vi "ULSIFD.vi"(0 "IFD in":refnum<class "IFD.lvclass">, 1 "ROI":cluster{"X1":sgl, "X2":sgl, "Y1":sgl, "Y2":sgl}={"X1"=0.0, "X2"=1.0, "Y1"=0.0, "Y2"=1.0}, 2 "General Info":T6={"CCD Model Num"="V10E", "Exposure time(ms)"=10.0, "Average"=1, "Boxcar"=0, "Pixel Count"=512, "Readout Mode"=enum."FVB", "Spec Mode"=enum."Wavelength(nm)", "Grating Groove"=1200, "Blaze"=500, "Data BG"=enum."No BG", "Ref BG"=enum."No BG", "Data Processed"=enum."No Ref", "Process Method"=enum."Not Selected", "Real Y"=0.0, "Real X"=0.0, "VSS"=0.0, "HSS"=0, "Step Length"=0}, 3 "Array Data":T5) -> (6 "IFD out":refnum<class "IFD.lvclass">)   [LabVIEW 2016]
uses:
  tiffInfo.ctl
  lib/Halloween/SaveTIFF/Class/IFD/IFD.lvclass
  lib/Halloween/SaveTIFF/Class/Tag/IFD_Tag.lvclass/IFD_Tag.ctl
  lib/Halloween/SaveTIFF/Class/Tag/IFD_Tag.lvclass
  lib/Halloween/SaveTIFF/Class/IFD/IFD.lvclass/IFD.ctl
panel:
  in  "Scan Rate(sample/sec)":dbl=1000.0 format="%#_13g"
  in  "Objective":u32=1
  in  "Scan Dimension":T1={"ROI"=enum."Rectangle", "Z layer count"=255, "Time Lapse"=enum."None"}
  in  "Scanner Component":T2={"Detector"=enum."Andor CCD", "Mover"=enum."Sigmakoki Stage"}
  in  "Settings Array":T3(array[cluster])
  in  "Hardware Model":T4={"Controller"=enum."SHOT-304", "X Stage"="", "Y Stage"="", "Z Stage"="", "R Stage"=""}
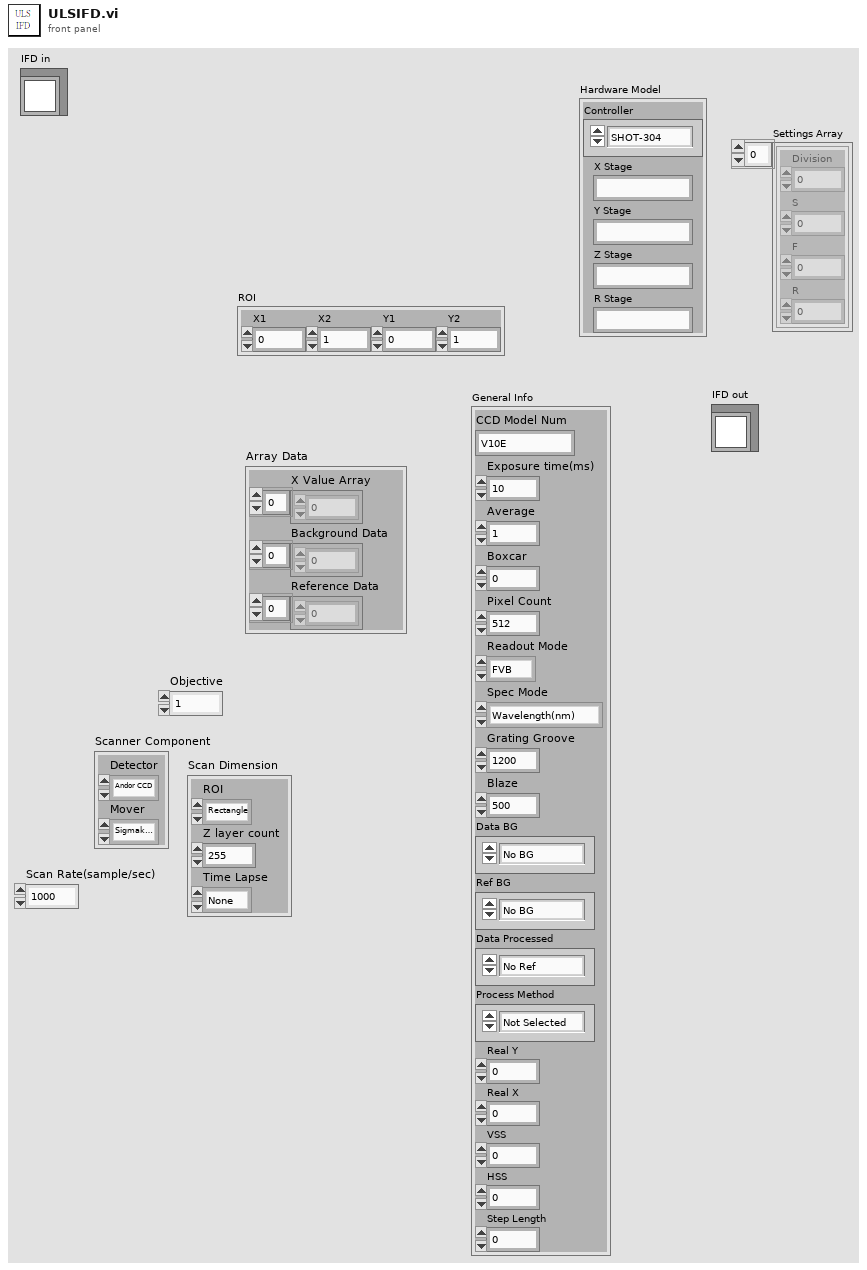
[diagram p1: front panel]
types:
  T1 = cluster{"ROI":enum8{"Undefined: No Ref", "Point", "Line", "Rectangle", "Square"}, "Z layer count":u8, "Time Lapse":enum8{"None", "Toe to Head", "Head to Head"}}
  T2 = cluster{"Detector":enum16{"Mightex BUF CCD", "PMT", "Andor CCD"}, "Mover":enum16{"None", "Galvo", "Sigmakoki Stage"}}
  T3 = cluster{"Division":u8, "S":u32, "F":u32, "R":u32}[]
  T4 = cluster{"Controller":enum32{"GSC-01(PAT)", "SHOT-102", "SHOT-302", "SHOT-602", "SHOT-702", "FINE-503", "SHOT-204", "SHOT-304"}, "X Stage":string, "Y Stage":string, "Z Stage":string, "R Stage":string}
  T5 = cluster{"X Value Array":sgl[], "Background Data":u16[], "Reference Data":u16[]}
  T6 = typedef "tiffInfo.ctl" = cluster{"CCD Model Num":string, "Exposure time(ms)":sgl, "Average":u8, "Boxcar":u8, "Pixel Count":u32, "Readout Mode":enum8{"FVB", "Multi Track", "Random Track", "Single Track", "2D"}, "Spec Mode":enum8{"Wavelength(nm)", "Wavenumber(/cm)"}, "Grating Groove":u16, "Blaze":u16, "Data BG":enum8{"No BG", "Not Subtracted", "Subtracted"}, "Ref BG":enum8{"No BG", "Not Subtracted", "Subtracted"}, "Data Processed":enum8{"No Ref", "Not Processed", "Processed"}, "Process Method":enum8{"Not Selected", "Absorption", "Transmission", "Subtraction"}, "Real Y":sgl, "Real X":sgl, "VSS":sgl, "HSS":u32, "Step Length":u32}
  T7 = enum16{"Undefined(DO NOT USE)", "U8", "ASCII", "U16", "U32", "RATIONAL", "I8", "Undefined 8 bit", "I16", "I32", "SRATIONAL", "SGL", "DBL"}
  T8 = enum16{"big-endian, network order", "native, host order", "little-endian"}
  T9 = enum8{"FVB", "Multi Track", "Random Track", "Single Track", "2D"}
  T10 = enum8{"Not Selected", "Absorption", "Transmission", "Subtraction"}
  T11 = enum32{"GSC-01(PAT)", "SHOT-102", "SHOT-302", "SHOT-602", "SHOT-702", "FINE-503", "SHOT-204", "SHOT-304"}
  T12 = cluster{"Data BG":enum8{"No BG", "Not Subtracted", "Subtracted"}, "Ref BG":enum8{"No BG", "Not Subtracted", "Subtracted"}, "Data Processed":enum8{"No Ref", "Not Processed", "Processed"}, "Process Method":enum8{"Not Selected", "Absorption", "Transmission", "Subtraction"}}
  T13 = cluster{"Spec Mode":enum8{"Wavelength(nm)", "Wavenumber(/cm)"}, "Average":u8, "Boxcar":u8, "Readout Mode":enum8{"FVB", "Multi Track", "Random Track", "Single Track", "2D"}}
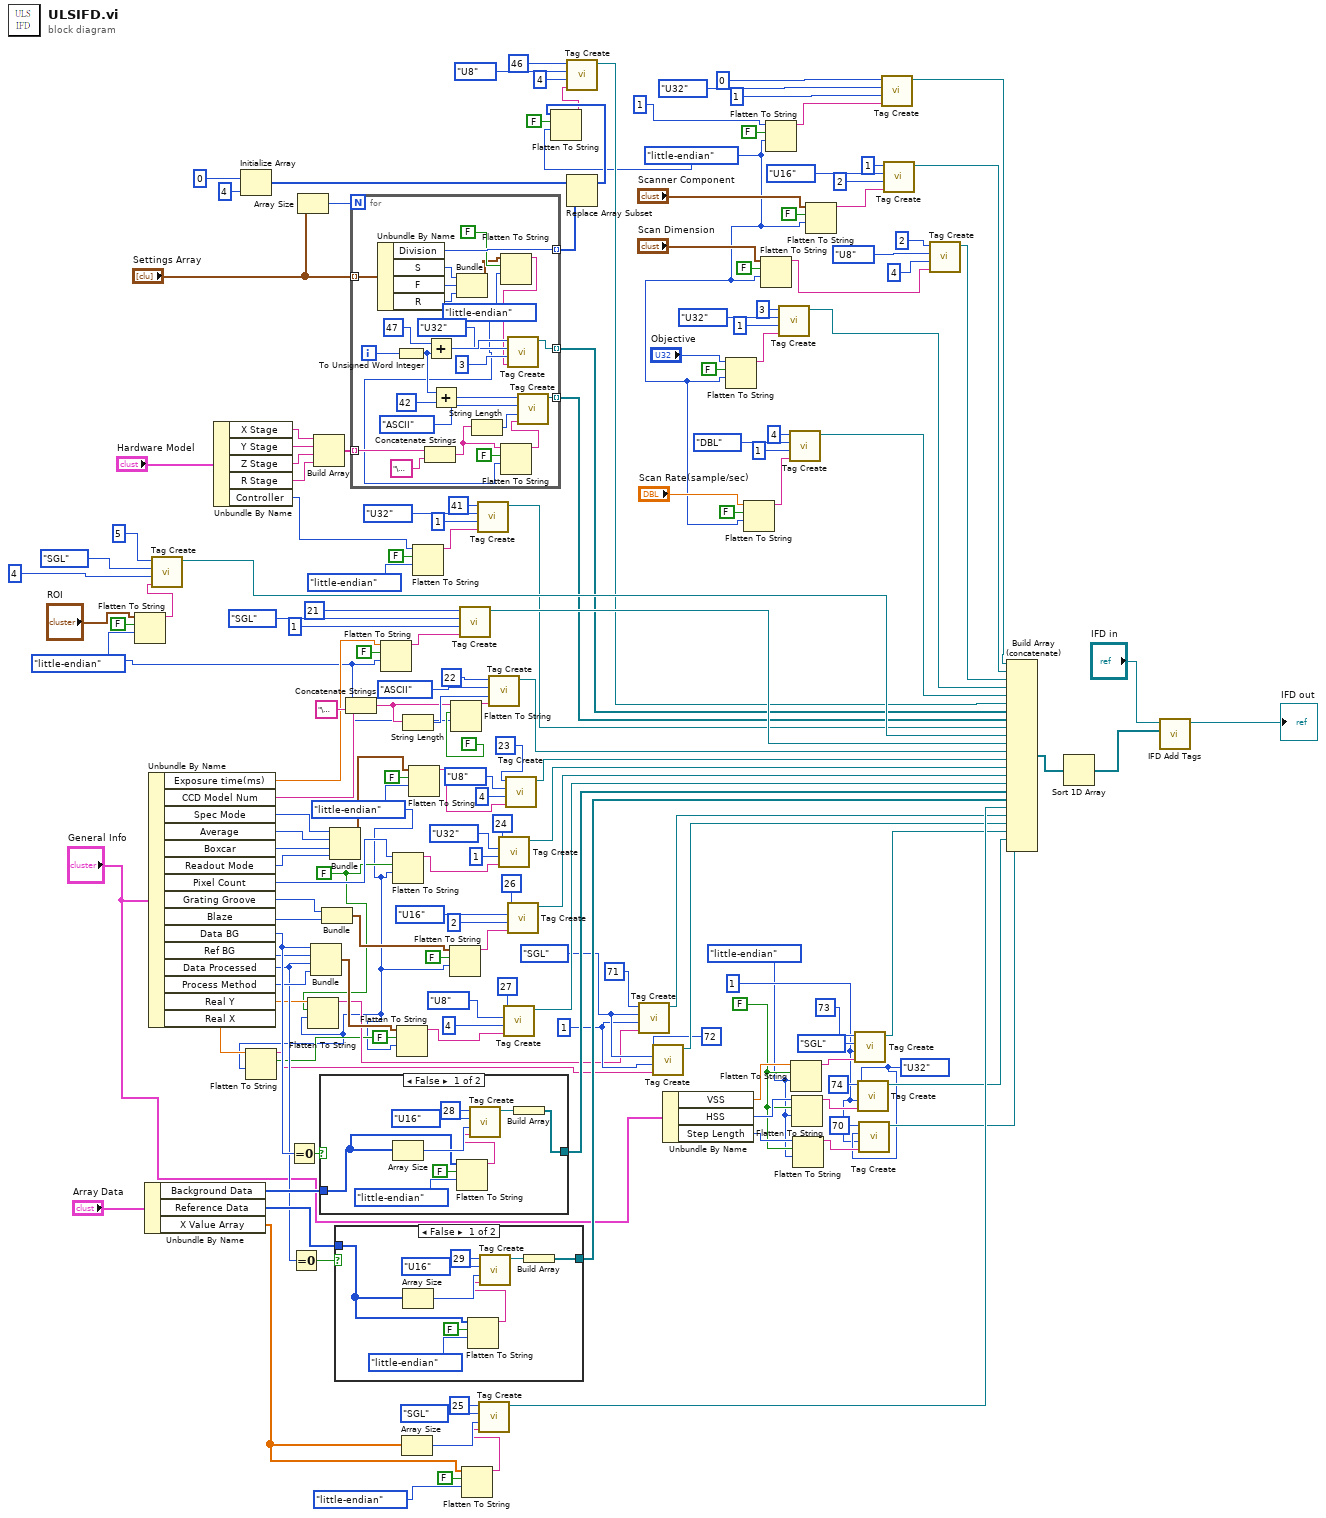
[diagram p0: block diagram]
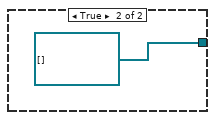
[diagram p2: hidden frame]
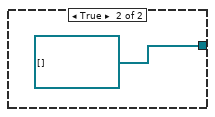
[diagram p3: hidden frame]
diagram:
  w6 = T7."U32" ("Data Type")
  w1 = T8."little-endian" ("byte order (0:big-endian, network order)")
  w2 = FALSE ("prepend array or string size? (T)")
  w5 = u32 1 ("Data Count")
  w29 = T7."SGL" ("Data Type")
  w28 = u32 1 ("Data Count")
  w20 = FALSE ("prepend array or string size? (T)")
  w24 = FALSE ("prepend array or string size? (T)")
  w43 = T8."little-endian" ("byte order (0:big-endian, network order)")
  w57 = T8."little-endian" ("byte order (0:big-endian, network order)")
  w19 = T8."little-endian" ("byte order (0:big-endian, network order)")
  n1 = Flatten To String(anything="ROI", prepend array or string size? (T)=FALSE, byte order (0:big-endian, network order)=w43) -> (data string=w50:string)  [unwired: 1 in, 2 out]
  n2 = Unbundle By Name("Array Data") -> ("Background Data"=w145:u16[], "Reference Data"=w142:u16[], "X Value Array"=w34:sgl[])
  n3 = Unbundle By Name("General Info") -> ("Exposure time(ms)"=w48:sgl, "CCD Model Num"=w164:string, "Spec Mode"=w130:enum8{"Wavelength(nm)", "Wavenumber(/cm)"}, "Average"=w129:u8, "Boxcar"=w128:u8, "Readout Mode"=w127:T9, "Pixel Count"=w42:u32, "Grating Groove"=w155:u16, "Blaze"=w154:u16, "Data BG"=w148:enum8{"No BG", "Not Subtracted", "Subtracted"}, "Ref BG"=w137:enum8{"No BG", "Not Subtracted", "Subtracted"}, "Data Processed"=w135:enum8{"No Ref", "Not Processed", "Processed"}, "Process Method"=w136:T10, "Real Y"=w25:sgl, "Real X"=w22:sgl)
  n4 = call "Tag Create.vi"("Data"=w50, "Data Count"=u32 4, "Data Type"=T7."SGL", "Tag ID"=u16 5) -> ("IFD_Tag out"=w122:refnum<class "IFD_Tag.lvclass">)  [unwired: 7 in]
  n5 = Unbundle By Name("Hardware Model") -> ("X Stage"=w120:string, "Y Stage"=w119:string, "Z Stage"=w118:string, "R Stage"=w117:string, "Controller"=w55:T11)
  n6 = Initialize Array(u8 0, 4 ("dimension size")) -> (w105:u8[])
  n7 = Flatten To String(anything=w22, prepend array or string size? (T)=w20, byte order (0:big-endian, network order)=w19) -> (data string=w21:string)  [unwired: 1 in, 2 out]
  n8 = Equal To 0?(x=w148) -> (x = 0?=w146:bool)
  n9 = Equal To 0?(x=w135) -> (x = 0?=w143:bool)
  n10 = Array Size(array="Settings Array") -> (size(s)=w116:i32)
  n11 = Flatten To String(anything=w25, prepend array or string size? (T)=w24, byte order (0:big-endian, network order)=w19) -> (data string=w23:string)  [unwired: 1 in, 2 out]
  n12 = Bundle("Data BG"=w148, "Ref BG"=w137, "Data Processed"=w135, "Process Method"=w136) -> (w37:T12)  [unwired: 1 in]
  n13 = Build Array(w120, w119, w118, w117) -> (w114:string[])
  n14 = case shown="False" w146 {
    tunnel: [w183 refnum<class "IFD_Tag.lvclass">[] []] -> w147
    tunnel: w145 -> [w178 _]
    frame False {
      n15 = Array Size(array=w178) -> (size(s)=w180:i32)
      n16 = Flatten To String(anything=w178, prepend array or string size? (T)=FALSE, byte order (0:big-endian, network order)=T8."little-endian") -> (data string=w177:string)  [unwired: 1 in, 2 out]
      n17 = call "Tag Create.vi"("Data"=w177, "Data Count"=w180, "Data Type"=T7."U16", "Tag ID"=u16 28) -> ("IFD_Tag out"=w184:refnum<class "IFD_Tag.lvclass">)  [unwired: 7 in]
      n18 = Build Array(w184) -> (w183:refnum<class "IFD_Tag.lvclass">[])
    }
    frame True {
    }
  }
  n19 = Bundle("Grating Groove"=w155, "Blaze"=w154) -> (w39:cluster{"Grating Groove":u16, "Blaze":u16})  [unwired: 1 in]
  n20 = Bundle("Spec Mode"=w130, "Average"=w129, "Boxcar"=w128, "Readout Mode"=w127) -> (w77:T13)  [unwired: 1 in]
  n21 = case shown="False" w143 {
    tunnel: [w193 refnum<class "IFD_Tag.lvclass">[] []] -> w144
    tunnel: w142 -> [w188 _]
    frame False {
      n22 = Array Size(array=w188) -> (size(s)=w190:i32)
      n23 = Flatten To String(anything=w188, prepend array or string size? (T)=FALSE, byte order (0:big-endian, network order)=T8."little-endian") -> (data string=w187:string)  [unwired: 1 in, 2 out]
      n24 = call "Tag Create.vi"("Data"=w187, "Data Count"=w190, "Data Type"=T7."U16", "Tag ID"=u16 29) -> ("IFD_Tag out"=w194:refnum<class "IFD_Tag.lvclass">)  [unwired: 7 in]
      n25 = Build Array(w194) -> (w193:refnum<class "IFD_Tag.lvclass">[])
    }
    frame True {
    }
  }
  n26 = Concatenate Strings(w164, "\u0000") -> (w45:string)
  n27 = for {
    N: w116 -> [_]
    tunnel: "Settings Array" -> [w221] mode=indexing
    tunnel: w114 -> [w208] mode=indexing
    tunnel: [w213] -> w101 mode=indexing
    tunnel: [w205] -> w102 mode=indexing
    tunnel: [w203] -> w104 mode=indexing
    i -> [w204]
    w196 = T8."little-endian" ("byte order (0:big-endian, network order)")
    n28 = Unbundle By Name(w221) -> ("Division"=w203:u8, "S"=w217:u32, "F"=w218:u32, "R"=w216:u32)
    n29 = To Unsigned Word Integer(number=w204) -> (unsigned 16bit integer=w211:u16)
    n30 = Concatenate Strings(w208, "\u0000") -> (w198:string)
    n31 = Add(x=u16 47 ("Tag ID"), y=w211) -> (x+y=w219:u16)
    n32 = Add(x=w211, y=u16 42 ("Tag ID")) -> (x+y=w210:u16)
    n33 = Bundle("S"=w217, "F"=w218, "R"=w216) -> (w201:cluster{"S":u32, "F":u32, "R":u32})  [unwired: 1 in]
    n34 = String Length(string=w198) -> (length=w206:i32)
    n35 = Flatten To String(anything=w201, prepend array or string size? (T)=FALSE, byte order (0:big-endian, network order)=w196) -> (data string=w200:string)  [unwired: 1 in, 2 out]
    n36 = Flatten To String(anything=w198, prepend array or string size? (T)=FALSE, byte order (0:big-endian, network order)=w196) -> (data string=w197:string)  [unwired: 1 in, 2 out]
    n37 = call "Tag Create.vi"("Data"=w200, "Data Count"=u32 3, "Data Type"=T7."U32", "Tag ID"=w219) -> ("IFD_Tag out"=w213:refnum<class "IFD_Tag.lvclass">)  [unwired: 7 in]
    n38 = call "Tag Create.vi"("Data"=w197, "Data Count"=w206, "Data Type"=T7."ASCII", "Tag ID"=w210) -> ("IFD_Tag out"=w205:refnum<class "IFD_Tag.lvclass">)  [unwired: 7 in]
  }
  n39 = Flatten To String(anything=w48, prepend array or string size? (T)=FALSE, byte order (0:big-endian, network order)=w43) -> (data string=w47:string)  [unwired: 1 in, 2 out]
  n40 = Flatten To String(anything=w42, prepend array or string size? (T)=w24, byte order (0:big-endian, network order)=w19) -> (data string=w41:string)  [unwired: 1 in, 2 out]
  n41 = Flatten To String(anything=w37, prepend array or string size? (T)=w20, byte order (0:big-endian, network order)=w19) -> (data string=w36:string)  [unwired: 1 in, 2 out]
  n42 = Array Size(array=w34) -> (size(s)=w141:i32)
  n43 = String Length(string=w45) -> (length=w162:i32)
  n44 = Flatten To String(anything=w77, prepend array or string size? (T)=FALSE, byte order (0:big-endian, network order)=w19) -> (data string=w76:string)  [unwired: 1 in, 2 out]
  n45 = Flatten To String(anything=w55, prepend array or string size? (T)=FALSE, byte order (0:big-endian, network order)=T8."little-endian") -> (data string=w54:string)  [unwired: 1 in, 2 out]
  n46 = Flatten To String(anything=w39, prepend array or string size? (T)=FALSE, byte order (0:big-endian, network order)=w19) -> (data string=w38:string)  [unwired: 1 in, 2 out]
  n47 = Flatten To String(anything=w45, prepend array or string size? (T)=FALSE, byte order (0:big-endian, network order)=w43) -> (data string=w44:string)  [unwired: 1 in, 2 out]
  n48 = call "Tag Create.vi"("Data"=w47, "Data Count"=u32 1, "Data Type"=T7."SGL", "Tag ID"=u16 21) -> ("IFD_Tag out"=w175:refnum<class "IFD_Tag.lvclass">)  [unwired: 7 in]
  n49 = Flatten To String(anything=w34, prepend array or string size? (T)=FALSE, byte order (0:big-endian, network order)=T8."little-endian") -> (data string=w33:string)  [unwired: 1 in, 2 out]
  n50 = call "Tag Create.vi"("Data"=w54, "Data Count"=u32 1, "Data Type"=T7."U32", "Tag ID"=u16 41) -> ("IFD_Tag out"=w103:refnum<class "IFD_Tag.lvclass">)  [unwired: 7 in]
  n51 = call "Tag Create.vi"("Data"=w33, "Data Count"=w141, "Data Type"=T7."SGL", "Tag ID"=u16 25) -> ("IFD_Tag out"=w138:refnum<class "IFD_Tag.lvclass">)  [unwired: 7 in]
  n52 = call "Tag Create.vi"("Data"=w44, "Data Count"=w162, "Data Type"=T7."ASCII", "Tag ID"=u16 22) -> ("IFD_Tag out"=w171:refnum<class "IFD_Tag.lvclass">)  [unwired: 7 in]
  n53 = call "Tag Create.vi"("Data"=w41, "Data Count"=u32 1, "Data Type"=T7."U32", "Tag ID"=u16 24) -> ("IFD_Tag out"=w169:refnum<class "IFD_Tag.lvclass">)  [unwired: 7 in]
  n54 = call "Tag Create.vi"("Data"=w36, "Data Count"=u32 4, "Data Type"=T7."U8", "Tag ID"=u16 27) -> ("IFD_Tag out"=w167:refnum<class "IFD_Tag.lvclass">)  [unwired: 7 in]
  n55 = call "Tag Create.vi"("Data"=w76, "Data Count"=u32 4, "Data Type"=T7."U8", "Tag ID"=u16 23) -> ("IFD_Tag out"=w170:refnum<class "IFD_Tag.lvclass">)  [unwired: 7 in]
  n56 = call "Tag Create.vi"("Data"=w38, "Data Count"=u32 2, "Data Type"=T7."U16", "Tag ID"=u16 26) -> ("IFD_Tag out"=w168:refnum<class "IFD_Tag.lvclass">)  [unwired: 7 in]
  n57 = Replace Array Subset(array=w105, new element=w104) -> (w59:u8[])  [unwired: 1 in]
  n58 = Flatten To String(anything=w59, prepend array or string size? (T)=FALSE, byte order (0:big-endian, network order)=w57) -> (data string=w58:string)  [unwired: 1 in, 2 out]
  n59 = call "Tag Create.vi"("Data"=w58, "Data Count"=u32 4, "Data Type"=T7."U8", "Tag ID"=u16 46) -> ("IFD_Tag out"=w100:refnum<class "IFD_Tag.lvclass">)  [unwired: 7 in]
  n60 = call "Tag Create.vi"("Data"=w23, "Data Count"=w28, "Data Type"=w29, "Tag ID"=u16 71) -> ("IFD_Tag out"=w30:refnum<class "IFD_Tag.lvclass">)  [unwired: 7 in]
  n61 = call "Tag Create.vi"("Data"=w21, "Data Count"=w28, "Data Type"=w29, "Tag ID"=u16 72) -> ("IFD_Tag out"=w27:refnum<class "IFD_Tag.lvclass">)  [unwired: 7 in]
  n62 = Unbundle By Name("General Info") -> ("VSS"=w13:sgl, "HSS"=w12:u32, "Step Length"=w3:u32)
  n63 = Flatten To String(anything="Objective", prepend array or string size? (T)=FALSE, byte order (0:big-endian, network order)=w57) -> (data string=w64:string)  [unwired: 1 in, 2 out]
  n64 = Flatten To String(anything="Scan Rate(sample/sec)", prepend array or string size? (T)=FALSE, byte order (0:big-endian, network order)=w57) -> (data string=w61:string)  [unwired: 1 in, 2 out]
  n65 = Flatten To String(anything="Scan Dimension", prepend array or string size? (T)=FALSE, byte order (0:big-endian, network order)=w57) -> (data string=w67:string)  [unwired: 1 in, 2 out]
  n66 = Flatten To String(anything=u32 1, prepend array or string size? (T)=FALSE, byte order (0:big-endian, network order)=w57) -> (data string=w73:string)  [unwired: 1 in, 2 out]
  n67 = call "Tag Create.vi"("Data"=w64, "Data Count"=u32 1, "Data Type"=T7."U32", "Tag ID"=u16 3) -> ("IFD_Tag out"=w83:refnum<class "IFD_Tag.lvclass">)  [unwired: 7 in]
  n68 = call "Tag Create.vi"("Data"=w61, "Data Count"=u32 1, "Data Type"=T7."DBL", "Tag ID"=u16 4) -> ("IFD_Tag out"=w84:refnum<class "IFD_Tag.lvclass">)  [unwired: 7 in]
  n69 = Flatten To String(anything=w13, prepend array or string size? (T)=w2, byte order (0:big-endian, network order)=w1) -> (data string=w16:string)  [unwired: 1 in, 2 out]
  n70 = Flatten To String(anything=w12, prepend array or string size? (T)=w2, byte order (0:big-endian, network order)=w1) -> (data string=w11:string)  [unwired: 1 in, 2 out]
  n71 = Flatten To String(anything=w3, prepend array or string size? (T)=w2, byte order (0:big-endian, network order)=w1) -> (data string=w8:string)  [unwired: 1 in, 2 out]
  n72 = Flatten To String(anything="Scanner Component", prepend array or string size? (T)=FALSE, byte order (0:big-endian, network order)=w57) -> (data string=w70:string)  [unwired: 1 in, 2 out]
  n73 = call "Tag Create.vi"("Data"=w16, "Data Count"=w5, "Data Type"=T7."SGL", "Tag ID"=u16 73) -> ("IFD_Tag out"=w15:refnum<class "IFD_Tag.lvclass">)  [unwired: 7 in]
  n74 = call "Tag Create.vi"("Data"=w11, "Data Count"=w5, "Data Type"=w6, "Tag ID"=u16 74) -> ("IFD_Tag out"=w10:refnum<class "IFD_Tag.lvclass">)  [unwired: 7 in]
  n75 = call "Tag Create.vi"("Data"=w8, "Data Count"=w5, "Data Type"=w6, "Tag ID"=u16 70) -> ("IFD_Tag out"=w7:refnum<class "IFD_Tag.lvclass">)  [unwired: 7 in]
  n76 = call "Tag Create.vi"("Data"=w73, "Data Count"=u32 1, "Data Type"=T7."U32", "Tag ID"=u16 0) -> ("IFD_Tag out"=w80:refnum<class "IFD_Tag.lvclass">)  [unwired: 7 in]
  n77 = call "Tag Create.vi"("Data"=w70, "Data Count"=u32 2, "Data Type"=T7."U16", "Tag ID"=u16 1) -> ("IFD_Tag out"=w81:refnum<class "IFD_Tag.lvclass">)  [unwired: 7 in]
  n78 = call "Tag Create.vi"("Data"=w67, "Data Count"=u32 4, "Data Type"=T7."U8", "Tag ID"=u16 2) -> ("IFD_Tag out"=w82:refnum<class "IFD_Tag.lvclass">)  [unwired: 7 in]
  n79 = Build Array (concatenate)(w80, w81, w82, w83, w84, w100, w101, w102, w103, w122, w175, w171, w170, w169, w168, w167, w147, w144, w138, w30, w27, w15, w10, w7) -> (w132:refnum<class "IFD_Tag.lvclass">[])
  n80 = Sort 1D Array(array=w132) -> (sorted array=w131:refnum<class "IFD_Tag.lvclass">[])
  n81 = call "IFD Add Tags.vi"("Tag(s)"=w131, "IFD in"="IFD in") -> ("IFD out"=→"IFD out":refnum<class "IFD.lvclass">)  [unwired: 8 in, 1 out]
